vi "Index.vi"(8 "error in (no error)":errorcluster, 10 "Index":i32, 11 "Waveform Array in":refnum<class "Waveform Array.lvclass">) -> (0 "error out":errorcluster, 3 "Indexed element":refnum<class "Generic Data.lvclass">)   [LabVIEW 2020, in "Data.lvlib" / "Waveform Array.lvclass"]
doc: "Index an element from 'Generic Data in'.\nThis implementation returns a generic Waveform class with the indexed Waveform."
uses:
  Waveform Array.lvclass
  Generic Data.lvclass
  Waveform Array.lvclass/Waveform Array.ctl
  Waveform/Waveform.lvclass/Waveform.ctl
  Waveform/Waveform.lvclass
  C:/Users/Henri/OneDrive/LabVIEW/Framework/Data/Generic Data/Generic Data.lvclass
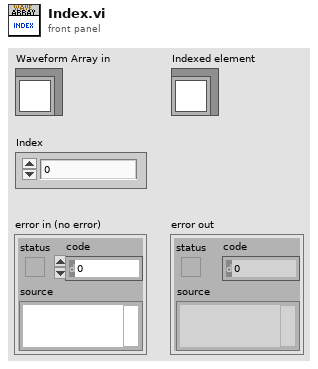
[diagram p1: front panel]
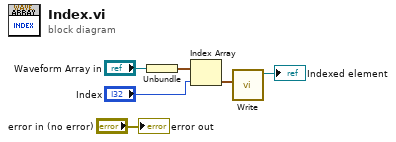
[diagram p0: block diagram]
diagram:
  n1 = Unbundle("Waveform Array in") -> (w5:waveform(dbl)[])
  n2 = Index Array(array=w5, index="Index") -> (element=w2:waveform(dbl))
  n3 = call "Write.vi"("Waveform"=w2) -> ("Waveform out"=→"Indexed element":refnum<class "Waveform.lvclass">)  [unwired: 10 in]
  "error out" <- "error in (no error)"
